vi "AnalogCNTL_Dakota3ch.vi"() -> ()   [LabVIEW 2015]
uses:
  <userlib>/caLab/Private/Put_DBL-1D_PV-1D.vi
  <vilib>/addons/control/pid/pid.llb/PID (DBL).vi
  <userlib>/caLab/Private/Get_PV-1D.vi
  <vilib>/addons/control/pid/NI_PID_pid.lvlib
  <vilib>/Analysis/NI_AALPro.lvlib
panel:
  out "APX:V7_SOP":bool
  out "APX:V7_SCL":bool
  in  "Gas_out_min_LIM":dbl min=0.0 max=1.0 step=0.02 format="%_3g"
  out "Error out":errorcluster
  out "APX:HPC":dbl format="%#_3g"
  out "APX:CellIn_MV":dbl
  out "APX:CellIn_MV2":dbl
  out "APX:CellIn_MV3":dbl
  out "Open 3":bool
  in  "Gas_in_min_LIM 3":dbl min=0.0 max=0.3 step=0.02 format="%_3g"
  in  "Gas_in_max_LIM 3":dbl min=0.0 max=2.0 step=0.02 format="%_3g"
  out "APX:CellIn_RV3":dbl(slide) scale=0.3..0.8
  out "slope OK":bool
  in  "slope loop":u8=15 min=10 max=30 step=1
  in  "Inlet2 offset":dbl
  out "APX:CellPressureState":u32
  in  "Threshold":dbl format="%#_13g"
  out "Inlet More":bool
  out "Open 2":bool
  in  "Gas_in_min_LIM 2":dbl min=0.0 max=0.3 step=0.02 format="%_3g"
  in  "Gas_in_max_LIM 2":dbl min=0.0 max=2.0 step=0.02 format="%_3g"
  out "APX:CellIn_RV2":dbl(slide) scale=0.3..0.8
  out "APX:CellOut_MV":dbl
  out "APX:OmniaxZ Failure":bool
  out "APX:CellMode":dbl
  out "APX:OmniaxZ":dbl
  out "APX:CellMode":bool
  out "PID_P":dbl format="%_4g"
  out "HPC Pressure Failure":bool
  out "HPC Turbo failure":bool
  out "<1.3":bool
  out "<2":bool
  out "OpenEx":bool
  out "APX:GAS":dbl format="%.2f"
  out "slope":dbl
  out "Open 1":bool
  in  "Inlet Mode":u16(ring) items=["Close", "Open", "Auto"]
  out "APX:CellIn_RV":sgl(slide)=0.8 min=0.3 max=0.8 step=0.05 scale=0.3..0.8
  out "Status":bool
  out "CellMode":u16
  out "Gas_out_max":dbl
  out "Period":i32
  out "Open Period":i32
  in  "Gas_in_min_LIM":dbl min=0.0 max=0.3 step=0.02 format="%_3g"
  in  "Gain":dbl=1.0 min=1.0 max=50.0 step=1.0 format="%_3g"
  in  "Gas_in_max_LIM":dbl=0.85 min=0.0 max=0.9 step=0.02 format="%_3g"
  in  "PID_D":dbl min=0.0 max=5.0 step=0.02 format="%_3g"
  in  "PID_I":dbl=0.5 min=0.005 max=5.0 step=0.02 format="%_3g"
  in  "PID_P_base":dbl=1.0 min=0.005 max=5.0 step=0.02 format="%_3g"
  in  "APX:CellPressure_RV":dbl=0.05 min=0.001 max=5.0 step=0.001 format="%.3f"
  out "PID_OC":dbl format="%.2f"
  out "PID dt out (s)":dbl format="%.3f"
  out "CellPressure":dbl(graph)
  in  "Exhasuet Mode":u16(ring) items=["Close", "Open", "Auto"]
  out "APX:AP1":dbl format="%#_3g"
  out "Outlet":sgl(slide)=2.0 min=0 max=5 step=0.05 scale=0.0..5.0
  out "APX:CellPressure_PV":dbl format="%_5g"
  in  "stop":bool
  # "Red LED ->\nClose-Close"
  # "if P>0.1 Period=Px100"
  # "Red LED ->\nClose-Open"
  # "Mk-II CH3"
  # "Ver 2023.12"
  # "0:Evacuate\n1: Auto-Auto\n2: Man-Man\n3: Man-Auto\n4: Auto-Man"
  # "Dakota 100000 sccm"
  # "8E-7 torr"
  # "record(ao, \"APX:CellIn_RV\")\n{\n    field(DESC, \"Double input without range infos\")\n    field(EGU, \"NA\")\n    field(PINI, \"YES\")\n}\nrecord(ao, \"APX:CellOut_RV\")\n{\n    field(DESC, \"Double input without range infos\")\n    field(EGU, \"NA\")\n    field(PINI, \"YES\")\n}\nrecord(ao, \"APX:CellIn_MV\")\n{\n    field(DESC, \"Double input without range infos\")\n    field(EGU, \"NA\")\n    field(PINI, \"YES\")\n}\nrecord(ao, \"APX:CellOut_MV\")\n{\n    field(DESC, \"Double input without range infos\")\n    field(EGU, \"NA\")\n    field(PINI, \"YES\")"
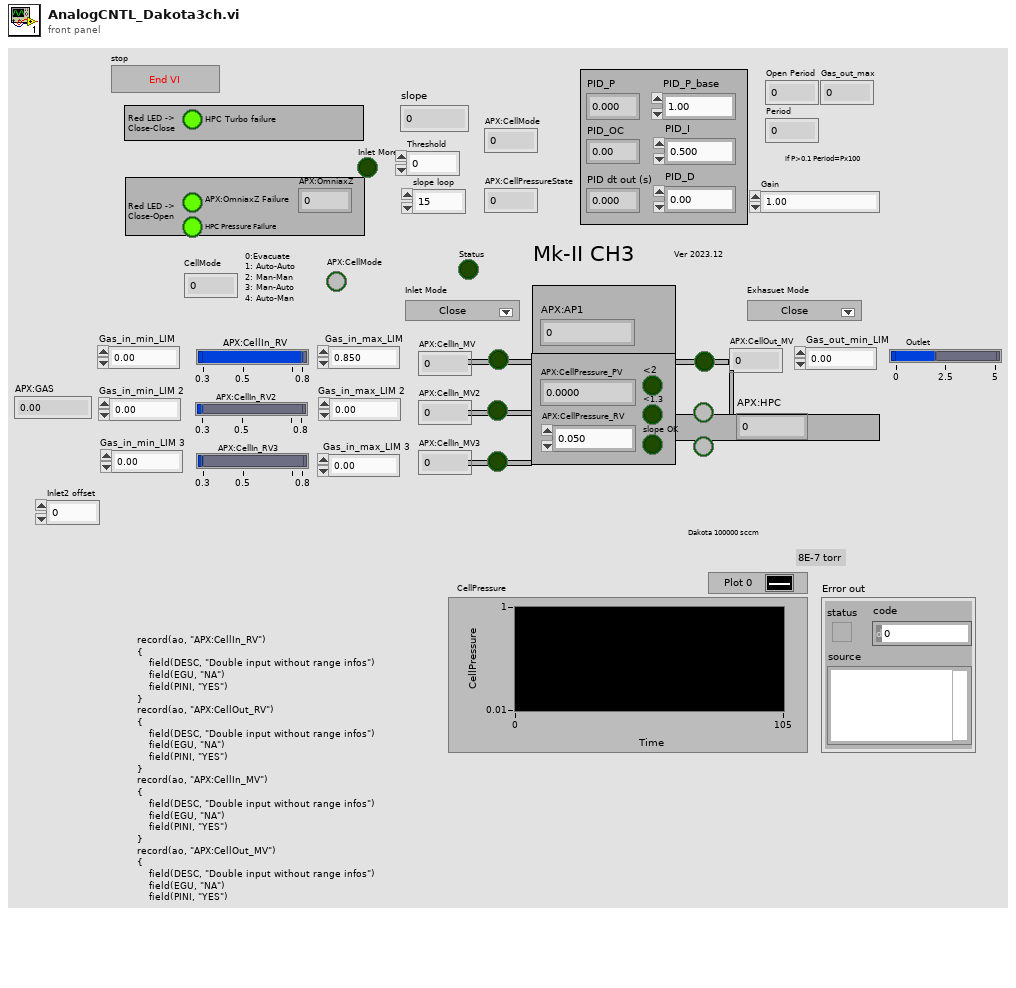
[diagram p1: front panel]
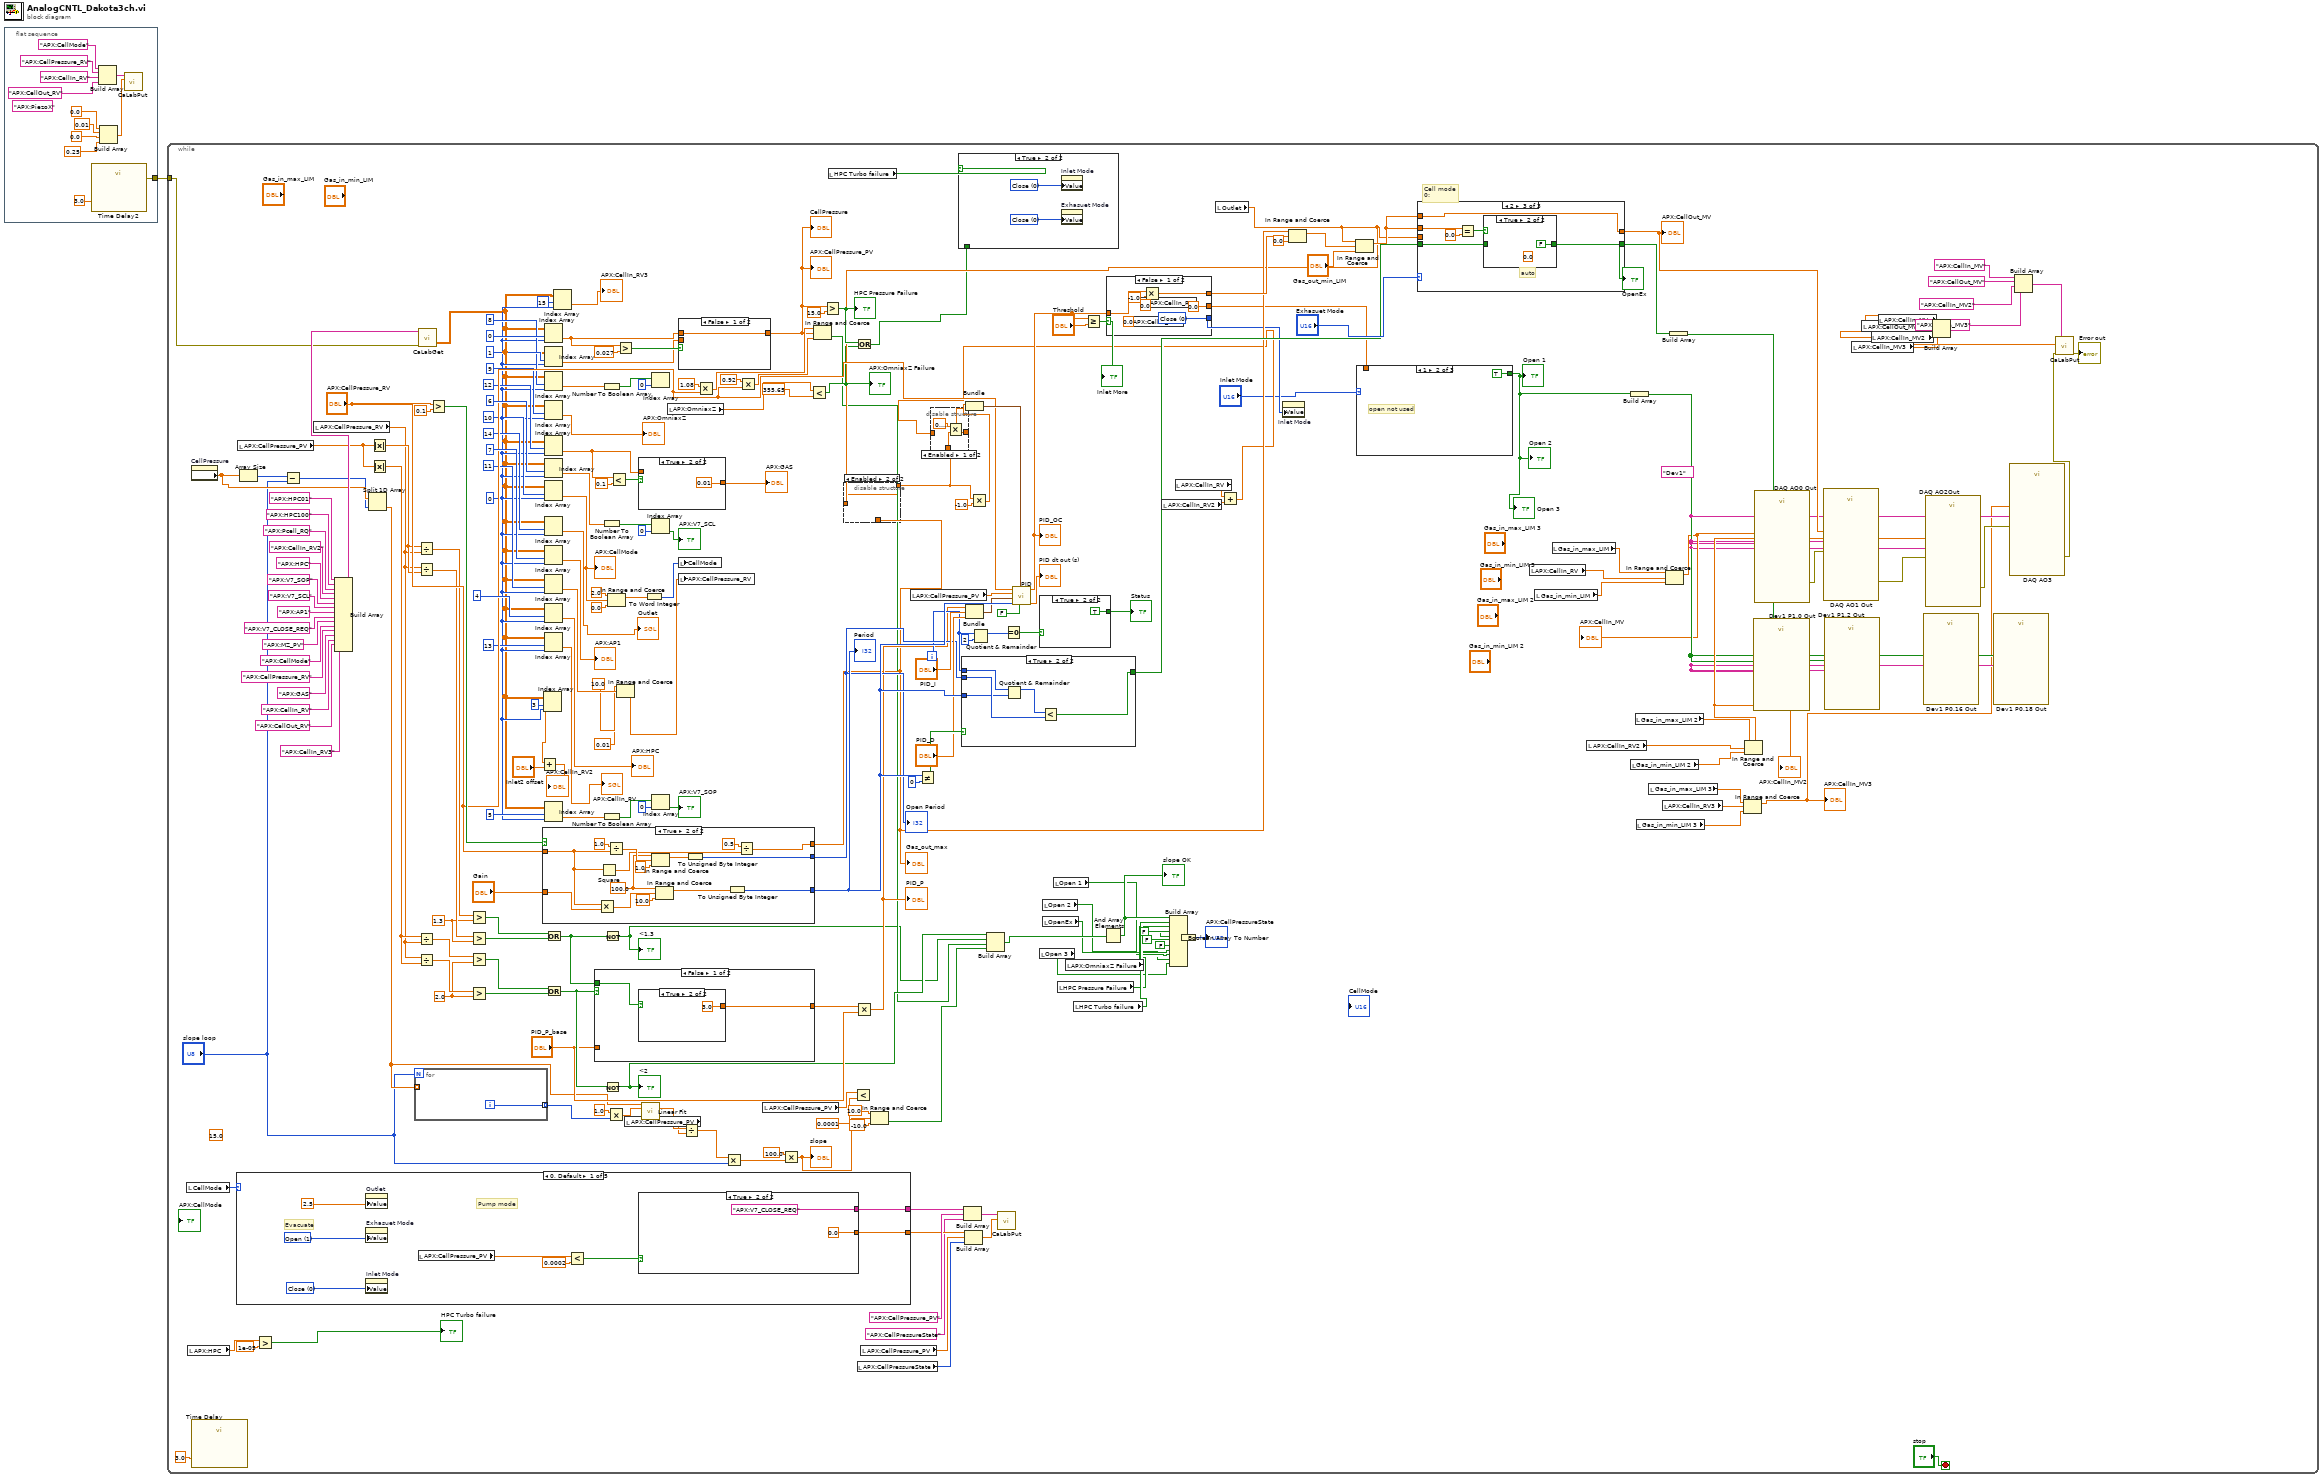
[diagram p0: block diagram]
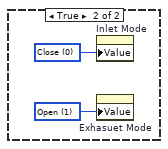
[diagram p6: hidden frame]
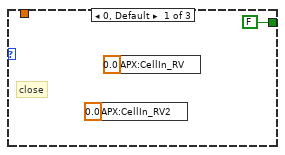
[diagram p7: hidden frame]
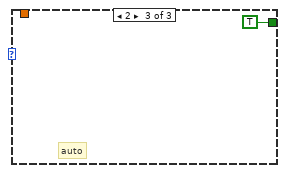
[diagram p8: hidden frame]
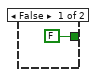
[diagram p9: hidden frame]
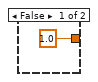
[diagram p10: hidden frame]
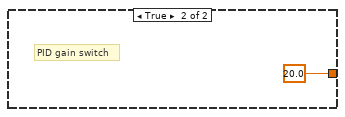
[diagram p11: hidden frame]
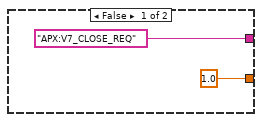
[diagram p12: hidden frame]
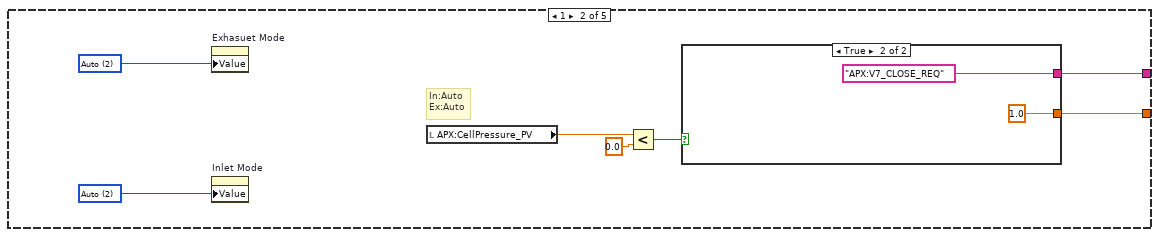
[diagram p13: hidden frame]
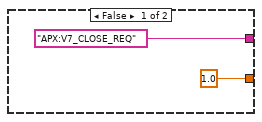
[diagram p14: hidden frame]
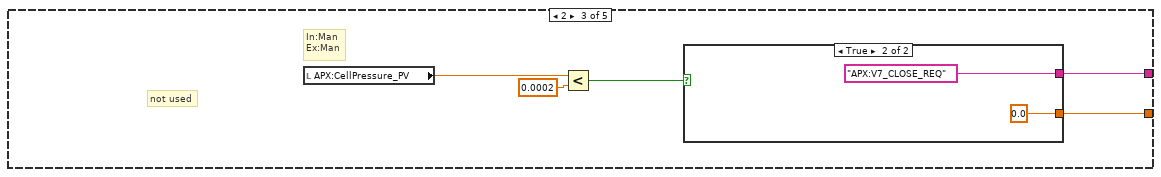
[diagram p15: hidden frame]
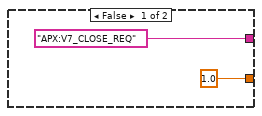
[diagram p16: hidden frame]
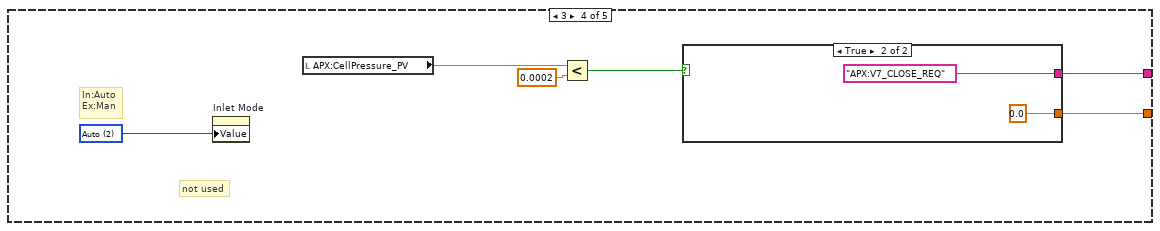
[diagram p17: hidden frame]
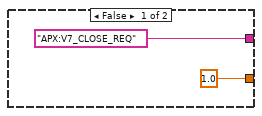
[diagram p18: hidden frame]
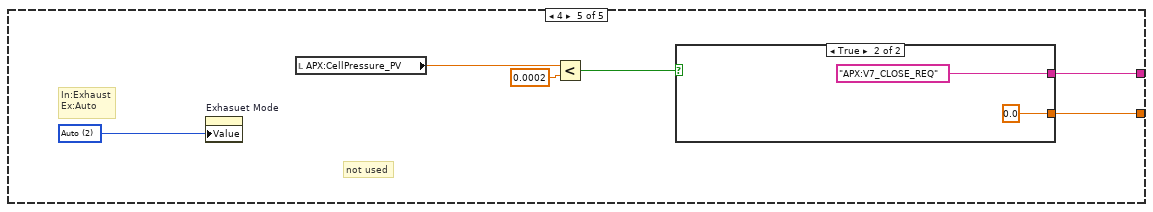
[diagram p19: hidden frame]
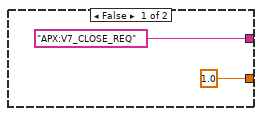
[diagram p20: hidden frame]
diagram:
  n1 = flat-sequence {
    tunnel: [w7] -> w1
    frame #0 {
      (unwired) "APX:PiezoX"
      n2 = call "Time Delay2"("Delay Time (s)"=3.0) -> ("error out"=w7:errorcluster)  [unwired: 10 in]
      n3 = Build Array("APX:CellMode", "APX:CellPressure_RV", "APX:CellIn_RV", "APX:CellOut_RV") -> (w11:string[])
      n4 = Build Array(0.0 ("element"), 0.01 ("element"), 0.0 ("element"), 0.25 ("element")) -> (w9:dbl[])
      n5 = call-poly <userlib>:"CaLabPut.vi"("Values"=w9, "PV Names"=w11) -> ()  [unwired: 6 in, 4 out]
    }
  }
  n6 = while {
    tunnel: w1 -> [w121]
    i -> [w176]
    stop <- "stop" stop-if-true
    w149 = 1.3 ("y")
    w158 = 2.0 ("y")
    (unwired) 15.0 ("y")
    w45 = 0 ("index (col)")
    w29 = tag "Dev1" ("device name")
    # "Cell mode \n0:"
    n7 = local read "CellMode"() -> (w111:u16)
    n8 = local read "APX:HPC"() -> (w139:dbl)
    n9 = property on="CellPressure" class="WFChart (strict)"() -> ("History Data"=w171:dbl[])  [unwired: 2 in, 2 out]
    n10 = call "Time Delay"("Delay Time (s)"=3.0) -> ()  [unwired: 10 in, 1 out]
    n11 = case shown="0, Default" w111 {
      tunnel: [w272 w283 w292 w302 w312] -> w127
      tunnel: [w271 w282 w291 w301 w311] -> w126
      frame 0, Default {
        w269 = u16 1 items=["Close", "Open", "Auto"] ("Exhasuet Mode")
        w270 = u16 0 items=["Close", "Open", "Auto"] ("Inlet Mod")
        # "Pump mode"
        # "Evacuate"
        n12 = property on="Outlet" class="Slide (strict)"("Value"=sgl 2.5 ("Exhaust")) -> ()  [unwired: 2 in, 2 out]
        n13 = property on="Exhasuet Mode" class="Ring (strict)"("Value"=w269) -> ()  [unwired: 2 in, 2 out]
        n14 = property on="Inlet Mode" class="Ring (strict)"("Value"=w270) -> ()  [unwired: 2 in, 2 out]
        n15 = local read "APX:CellPressure_PV"() -> (w267:dbl)
        n16 = Less?(x=w267, y=0.0002) -> (x < y?=w273:bool)
        n17 = case shown="True" w273 {
          tunnel: ["APX:V7_CLOSE_REQ" ("PV Name") "APX:V7_CLOSE_REQ" ("PV Name")] -> w272
          tunnel: [1.0 ("Value") 0.0 ("Value")] -> w271
          frame False {
          }
          frame True {
          }
        }
      }
      frame 1 {
        w280 = u16 2 items=["Close", "Open", "Auto"] ("Inlet Mod")
        w281 = u16 2 items=["Close", "Open", "Auto"] ("Exhasuet Mode")
        # "In:Auto\nEx:Auto"
        n18 = property on="Exhasuet Mode" class="Ring (strict)"("Value"=w281) -> ()  [unwired: 2 in, 2 out]
        n19 = property on="Inlet Mode" class="Ring (strict)"("Value"=w280) -> ()  [unwired: 2 in, 2 out]
        n20 = local read "APX:CellPressure_PV"() -> (w279:dbl)
        n21 = Less?(x=w279, y=0.0) -> (x < y?=w284:bool)
        n22 = case shown="True" w284 {
          tunnel: ["APX:V7_CLOSE_REQ" ("PV Name") "APX:V7_CLOSE_REQ" ("PV Name")] -> w283
          tunnel: [1.0 ("Value") 1.0 ("Value")] -> w282
          frame False {
          }
          frame True {
          }
        }
      }
      frame 2 {
        # "not used"
        # "In:Man\nEx:Man"
        n23 = local read "APX:CellPressure_PV"() -> (w290:dbl)
        n24 = Less?(x=w290, y=0.0002) -> (x < y?=w293:bool)
        n25 = case shown="True" w293 {
          tunnel: ["APX:V7_CLOSE_REQ" ("PV Name") "APX:V7_CLOSE_REQ" ("PV Name")] -> w292
          tunnel: [1.0 ("Value") 0.0 ("Value")] -> w291
          frame False {
          }
          frame True {
          }
        }
      }
      frame 3 {
        w300 = u16 2 items=["Close", "Open", "Auto"] ("Exhasuet Mode")
        # "not used"
        # "In:Auto\nEx:Man"
        n26 = property on="Inlet Mode" class="Ring (strict)"("Value"=w300) -> ()  [unwired: 2 in, 2 out]
        n27 = local read "APX:CellPressure_PV"() -> (w299:dbl)
        n28 = Less?(x=w299, y=0.0002) -> (x < y?=w303:bool)
        n29 = case shown="True" w303 {
          tunnel: ["APX:V7_CLOSE_REQ" ("PV Name") "APX:V7_CLOSE_REQ" ("PV Name")] -> w302
          tunnel: [1.0 ("Value") 0.0 ("Value")] -> w301
          frame False {
          }
          frame True {
          }
        }
      }
      frame 4 {
        w310 = u16 2 items=["Close", "Open", "Auto"] ("Exhasuet Mode")
        # "not used"
        # "In:Exhaust\nEx:Auto"
        n30 = property on="Exhasuet Mode" class="Ring (strict)"("Value"=w310) -> ()  [unwired: 2 in, 2 out]
        n31 = local read "APX:CellPressure_PV"() -> (w309:dbl)
        n32 = Less?(x=w309, y=0.0002) -> (x < y?=w313:bool)
        n33 = case shown="True" w313 {
          tunnel: ["APX:V7_CLOSE_REQ" ("PV Name") "APX:V7_CLOSE_REQ" ("PV Name")] -> w312
          tunnel: [1.0 ("Value") 0.0 ("Value")] -> w311
          frame False {
          }
          frame True {
          }
        }
      }
    }
    n34 = local read "APX:CellPressure_PV"() -> (w145:dbl)
    n35 = Array Size(array=w171) -> (size(s)=w169:i32)
    n36 = Greater?(x=w139, y=1e-05) -> (0:→"HPC Turbo failure":bool)
    n37 = Subtract(x=w169, y="slope loop") -> (x-y=w170:i32)
    n38 = local read "APX:CellPressure_RV"() -> (w144:dbl)
    n39 = Build Array("APX:HPC01", "APX:HPC100", "APX:Pcell_RQ", "APX:CellIn_RV2", "APX:HPC", "APX:V7_SOP", "APX:V7_SCL", "APX:AP1", "APX:V7_CLOSE_REQ", "APX:MZ_PV", "APX:CellMode", "APX:CellPressure_RV", "APX:GAS" ("element"), "APX:CellIn_RV", "APX:CellOut_RV", "APX:CellIn_RV3") -> (w239:string[])
    n40 = Split 1D Array(array=w171, index=w170) -> (second subarray=w73:dbl[])  [unwired: 1 out]
    n41 = Absolute Value(x=w145) -> (abs(x)=w146:dbl)
    n42 = Absolute Value(x=w145) -> (abs(x)=w152:dbl)
    n43 = for {
      N: "slope loop" -> [_]
      tunnel: w73 -> [_] mode=indexing
      tunnel: [w254] -> w168 mode=indexing
      i -> [w254]
    }
    n44 = Divide(x=w146, y=w144) -> (x/y=w151:dbl)
    n45 = Divide(x=w144, y=w146) -> (x/y=w150:dbl)
    n46 = Divide(x=w152, y=w144) -> (x/y=w160:dbl)
    n47 = Divide(x=w144, y=w152) -> (x/y=w159:dbl)
    n48 = call-poly "CaLabGet.vi"("PV Names"=w239, "Error in (no error)"=w121) -> ("Value Array (number)"=w43:dbl[][])  [unwired: 7 in, 6 out]
    n49 = Greater?(x="APX:CellPressure_RV", y=0.1) -> (0:w207:bool)
    n50 = Greater?(x=w151, y=w149) -> (0:w148:bool)
    n51 = Greater?(x=w150, y=w149) -> (0:w147:bool)
    n52 = Greater?(x=w160, y=w158) -> (0:w157:bool)
    n53 = Greater?(x=w159, y=w158) -> (0:w156:bool)
    n54 = case shown="True" w207 {
      tunnel: "APX:CellPressure_RV" -> [_ w332]
      tunnel: [w330 w341] -> w206
      tunnel: "Gain" -> [_ w345]
      tunnel: [w330 w335] -> w188
      tunnel: [5.0 w333] -> w87
      frame False {
        w330 = 10
      }
      frame True {
        w338 = 100.0 ("upper limit")
        n55 = Multiply(x=w332, y=w345) -> (x*y=w343:dbl)
        n56 = Square(x=w332) -> (x^2=w331:dbl)
        n57 = Divide(x=1.0, y=w332) -> (x/y=w339:dbl)
        n58 = In Range and Coerce(upper limit=w338, x=w339, lower limit=1.0) -> (coerced(x)=w336:dbl)  [unwired: 1 out]
        n59 = In Range and Coerce(upper limit=w338, x=w343, lower limit=10.0) -> (coerced(x)=w342:dbl)  [unwired: 1 out]
        n60 = To Unsigned Byte Integer(number=w336) -> (unsigned 8bit integer=w335:u8)
        n61 = To Unsigned Byte Integer(number=w342) -> (unsigned 8bit integer=w341:u8)
        n62 = Divide(x=0.5, y=w331) -> (x/y=w333:dbl)
      }
    }
    "Open Period" <- w188
    "Period" <- w206
    "Gas_out_max" <- w87
    n63 = Index Array(array=w43, index (row)=3, index (col)=w45) -> (element=w53:dbl)
    n64 = Add(x=w53, y="Inlet2 offset") -> (x+y=→"APX:CellIn_RV2":dbl)
    n65 = Index Array(array=w43, index (row)=1 ("disabled index (col)"), index (col)=w45) -> (element=w233:dbl)
    n66 = Index Array(array=w43, index (row)=8, index (col)=w45) -> (element=w184:dbl)
    n67 = Index Array(array=w43, index (row)=9 ("disabled index (row)"), index (col)=w45) -> (element=→"APX:OmniaxZ":dbl)
    n68 = Index Array(array=w43, index (row)=6, index (col)=w45) -> (element=w221:dbl)
    n69 = Index Array(array=w43, index (row)=14 ("disabled index (row)"), index (col)=w45) -> (element=→"Outlet":dbl)
    n70 = Index Array(array=w43, index (row)=7, index (col)=w45) -> (element=→"APX:AP1":dbl)
    n71 = Index Array(array=w43, index (row)=11, index (col)=w45) -> (element=w119:dbl)
    n72 = Index Array(array=w43, index (row)=4, index (col)=w45) -> (element=→"APX:HPC":dbl)
    n73 = Index Array(array=w43, index (row)=13 ("disabled index (row)"), index (col)=w45) -> (element=→"APX:CellIn_RV":dbl)
    n74 = Index Array(array=w43, index (row)=5, index (col)=w45) -> (element=w220:dbl)
    n75 = Index Array(array=w43, index (row)=0 ("disabled index (col)"), index (col)=w45) -> (element=w232:dbl)
    n76 = Index Array(array=w43, index (row)=12, index (col)=w45) -> (element=w103:dbl)
    n77 = Index Array(array=w43, index (row)=10, index (col)=w45) -> (element=w110:dbl)
    "APX:CellMode" <- w110
    n78 = Or(x=w148, y=w147) -> (x .or. y?=w143:bool)
    n79 = Or(x=w157, y=w156) -> (x .or. y?=w155:bool)
    n80 = Index Array(array=w43, index (row)=15, index (col)=w45) -> (element=→"APX:CellIn_RV3":dbl)
    n81 = case shown="False" w155 {
      tunnel: "PID_P_base" -> [_ _]
      tunnel: w143 -> [w263 _]
      tunnel: [w262 20.0 ("y")] -> w140
      frame False {
        n82 = case shown="True" w263 {
          tunnel: [1.0 ("y") 3.0 ("y")] -> w262
          frame False {
          }
          frame True {
          }
        }
      }
      frame True {
        # "PID gain switch"
      }
    }
    n83 = Number To Boolean Array(number=w184) -> (Boolean array=w183:bool[])
    n84 = Number To Boolean Array(number=w221) -> (Boolean array=w219:bool[])
    n85 = Number To Boolean Array(number=w220) -> (Boolean array=w216:bool[])
    n86 = Not(x=w143) -> (.not. x?=w51:bool)
    "<1.3" <- w51
    n87 = Not(x=w155) -> (.not. x?=w60:bool)
    "<2" <- w60
    n88 = Multiply(x=1.0, y=w168) -> (x*y=w167:dbl[])
    n89 = In Range and Coerce(upper limit=2.0, x=w110, lower limit=0.0) -> (coerced(x)=w112:dbl)  [unwired: 1 out]
    n90 = Less?(x=w103, y=0.1) -> (x < y?=w104:bool)
    n91 = Greater?(x=w232, y=0.027) -> (0:w235:bool)
    n92 = In Range and Coerce(upper limit=10.0, x=w119, lower limit=0.01) -> (coerced(x)=w116:dbl)  [unwired: 1 out]
    n93 = local read "APX:CellPressure_PV"() -> (w71:dbl)
    n94 = case shown="True" w104 {
      tunnel: w103 -> [w247 _]
      tunnel: [w247 0.01] -> w102
      frame False {
      }
      frame True {
      }
    }
    "APX:GAS" <- w102
    n95 = call <vilib>:"Linear Fit.vi"("Y"=w73, "X"=w167) -> ("slope"=w172:dbl)  [unwired: 9 in, 4 out]
    n96 = To Word Integer(number=w112) -> (16bit integer=w113:i16)
    n97 = Index Array(array=w183, index=0) -> ()  [unwired: 1 out]
    n98 = Index Array(array=w219, index=0) -> (element=→"APX:V7_SCL":bool)
    n99 = Index Array(array=w216, index=0) -> (element=→"APX:V7_SOP":bool)
    n100 = local read "APX:OmniaxZ"() -> (w62:dbl)
    n101 = case shown="False" w235 {
      tunnel: w233 -> [_ w371]
      tunnel: [w370 w371] -> w135
      tunnel: w232 -> [w370 _]
      frame False {
      }
      frame True {
      }
    }
    "APX:CellPressure_PV" <- w135
    "CellPressure" <- w135
    n102 = local write "CellMode"(w113) -> ()
    n103 = local write "APX:CellPressure_RV"(w116) -> ()
    n104 = Divide(x=w172, y=w71) -> (x/y=w162:dbl)
    n105 = Multiply(x=1.08, y="APX:CellPressure_RV") -> (x*y=w194:dbl)
    n106 = Multiply(x=w162, y="slope loop") -> (x*y=w161:dbl)
    n107 = Multiply(x=0.92, y="APX:CellPressure_RV") -> (x*y=w195:dbl)
    n108 = local read "APX:CellPressure_PV"() -> (w153:dbl)
    n109 = Multiply(x=100.0, y=w161) -> (x*y=w165:dbl)
    "slope" <- w165
    n110 = Less?(x=w62, y=355.65) -> (x < y?=w61:bool)
    "APX:OmniaxZ Failure" <- w61
    n111 = In Range and Coerce(upper limit=w194, x=w135, lower limit=w195) -> (In Range?=w59:bool)  [unwired: 1 out]
    n112 = Greater?(x=w135, y=15.0) -> (0:w134:bool)
    "HPC Pressure Failure" <- w134
    n113 = local read "HPC Turbo failure"() -> (w65:bool)
    n114 = Less?(x=w153, y=0.0001) -> ()  [unwired: 1 out]
    n115 = Or(x=w134, y=w61) -> (x .or. y?=w64:bool)
    n116 = Multiply(x=w140, y="PID_P_base") -> (x*y=w142:dbl)
    "PID_P" <- w142
    n117 = local read "APX:CellPressureState"() -> (w108:u32)
    n118 = local read "APX:CellPressure_PV"() -> (w123:dbl)
    n119 = In Range and Coerce(upper limit=10.0, x=w165, lower limit=-10.0) -> (In Range?=w58:bool)  [unwired: 1 out]
    n120 = local read "APX:CellPressure_PV"() -> (w186:dbl)
    n121 = Not Equal?(x=w206, y=u8 0) -> (x != y?=w212:bool)
    n122 = case shown="True" w65 {
      tunnel: w64 -> [w249 _]
      frame False {
        n123 = case shown="False" w249 {
          frame False {
          }
          frame True {
            w250 = u16 1 items=["Close", "Open", "Auto"] ("Inlet Mod")
            w251 = u16 0 items=["Close", "Open", "Auto"] ("Exhasuet Mode")
            n124 = property on="Inlet Mode" class="Ring (strict)"("Value"=w251) -> ()  [unwired: 2 in, 2 out]
            n125 = property on="Exhasuet Mode" class="Ring (strict)"("Value"=w250) -> ()  [unwired: 2 in, 2 out]
          }
        }
      }
      frame True {
        w252 = u16 0 items=["Close", "Open", "Auto"] ("Inlet Mod")
        w253 = u16 0 items=["Close", "Open", "Auto"] ("Exhasuet Mode")
        n126 = property on="Inlet Mode" class="Ring (strict)"("Value"=w253) -> ()  [unwired: 2 in, 2 out]
        n127 = property on="Exhasuet Mode" class="Ring (strict)"("Value"=w252) -> ()  [unwired: 2 in, 2 out]
      }
    }
    n128 = case shown="True" w212 {
      tunnel: w176 -> [_ w369]
      tunnel: [FALSE w368] -> w173
      tunnel: w206 -> [_ w365]
      tunnel: w188 -> [_ w367]
      frame False {
      }
      frame True {
        n129 = Quotient & Remainder(x=w369, y=w365) -> (x-y*floor(x/y)=w366:i32)  [unwired: 1 out]
        n130 = Less?(x=w366, y=w367) -> (x < y?=w368:bool)
      }
    }
    n131 = Build Array(w127, "APX:CellPressure_PV", "APX:CellPressureState") -> (w124:string[])
    n132 = Build Array(w126, w123, w108) -> (w125:dbl[])
    n133 = Bundle(w142, "PID_I"="PID_I", "PID_D"="PID_D") -> (w202:cluster{dbl, "PID_I":dbl, "PID_D":dbl})  [unwired: 1 in]
    n134 = Quotient & Remainder(x=w176, y=2) -> (x-y*floor(x/y)=w179:i32)  [unwired: 1 out]
    n135 = Build Array(w60, w51, w59, w58) -> (w57:bool[])
    n136 = call-poly <userlib>:"CaLabPut.vi"("Values"=w125, "PV Names"=w124) -> ()  [unwired: 6 in, 4 out]
    n137 = Equal To 0?(x=w179) -> (x = 0?=w180:bool)
    n138 = case shown="True" w180 {
      tunnel: [FALSE ("Status") TRUE ("Status")] -> w177
      frame False {
      }
      frame True {
      }
    }
    "Status" <- w177
    n139 = local read "Open 3"() -> (w16:bool)
    n140 = local read "Open 2"() -> (w17:bool)
    n141 = local read "OpenEx"() -> (w19:bool)
    n142 = local read "Open 1"() -> (w18:bool)
    n143 = local read "HPC Pressure Failure"() -> (w23:bool)
    n144 = local read "APX:OmniaxZ Failure"() -> (w24:bool)
    n145 = local read "HPC Turbo failure"() -> (w25:bool)
    n146 = And Array Elements(Boolean array=w57) -> (logical AND=w47:bool)
    "slope OK" <- w47
    n147 = local read "APX:CellIn_RV2"() -> (w75:dbl)
    n148 = Build Array(w47, w25, w24, w23, FALSE ("element"), FALSE ("element"), FALSE ("element"), w19, w18, w17, w16) -> (w56:bool[])
    n149 = local read "APX:CellIn_RV"() -> (w74:sgl)
    n150 = Boolean Array To Number(Boolean array=w56) -> (number=→"APX:CellPressureState":u32)
    n151 = local read "Outlet"() -> (w70:sgl)
    n152 = disable-structure shown="Enabled" {
      disable-tunnel: w87 -> [w245 _]
      disable-tunnel: [w245 w246] -> w67
      disable-tunnel: w70 -> [_ w246]
      frame Disabled {
      }
      frame Enabled {
      }
    }
    n153 = Multiply(x=w67, y=-1.0) -> (x*y=w86:dbl)
    n154 = Add(x=w74, y=w75) -> (x+y=w69:dbl)
    n155 = disable-structure shown="Enabled" {
      disable-tunnel: w69 -> [_ _]
      disable-tunnel: [w243 _] -> w68
      disable-tunnel: w67 -> [w244 _]
      frame Enabled {
        n156 = Multiply(x=sgl 0.1, y=w244) -> (x*y=w243:sgl)
      }
      frame Disabled {
      }
    }
    n157 = Bundle(w86, w68) -> (w199:cluster{dbl, sgl})  [unwired: 1 in]
    n158 = call-poly <vilib>:"PID.vi"("reinitialize? (F)"=FALSE, "output range"=w199, "dt (s)"=w206, "PID gains"=w202, "process variable"=w186, "setpoint"="APX:CellPressure_RV") -> ("dt out (s)"=→"PID dt out (s)":dbl, "output"=w189:dbl)  [unwired: 4 in]
    "PID_OC" <- w189
    n159 = Greater Or Equal?(x=w189, y="Threshold") -> (x >= y?=w197:bool)
    "Inlet More" <- w197
    n160 = case shown="False" w197 {
      tunnel: [w324 0.0] -> w190
      tunnel: w189 -> [w325 w327]
      tunnel: [0.0 w327] -> w66
      tunnel: [w321 w326] -> w50
      frame False {
        w321 = u16 0 items=["Close", "Open", "Auto"] ("Inlet Mode")
        n161 = local write "APX:CellIn_RV2"(0.0 ("Inlet2")) -> ()
        n162 = local write "APX:CellIn_RV"(sgl 0.0 ("Inlet")) -> ()
        n163 = Multiply(x=w325, y=-1.0) -> (x*y=w324:dbl)
      }
      frame True {
        w326 = u16 2 items=["Close", "Open", "Auto"] ("Inlet Mode")
      }
    }
    n164 = property on="Inlet Mode" class="Ring (strict)"("Value"=w50) -> ()  [unwired: 2 in, 2 out]
    n165 = In Range and Coerce(upper limit=w87, x=w190, lower limit=0.0) -> (coerced(x)=w89:dbl)  [unwired: 1 out]
    n166 = In Range and Coerce(upper limit=w70, x=w89, lower limit="Gas_out_min_LIM") -> (coerced(x)=w88:dbl)  [unwired: 1 out]
    n167 = case shown="1" "Inlet Mode" {
      tunnel: [FALSE TRUE TRUE] -> w41
      tunnel: w66 -> [_ _ _]
      frame 0, Default {
        # "close"
        n168 = local write "APX:CellIn_RV2"(0.0 ("Inlet2")) -> ()
        n169 = local write "APX:CellIn_RV"(sgl 0.0 ("Inlet")) -> ()
      }
      frame 1 {
        # "open not used"
      }
      frame 2 {
        # "auto"
      }
    }
    "Open 1" <- w41
    "Open 2" <- w41
    "Open 3" <- w41
    n170 = case shown="2" "Exhasuet Mode" {
      tunnel: w173 -> [_ w351 w357]
      tunnel: [0.0 2.5 ("y") w361] -> w175
      tunnel: w88 -> [_ _ w361]
      tunnel: w88 -> [_ _ w360]
      tunnel: w70 -> [_ w349 _]
      tunnel: [FALSE w350 w356] -> w90
      frame 0, Default {
        # "Close"
      }
      frame 1 {
        # "open"
        n171 = Equal?(x=w349, y=0.0) -> (x = y?=w352:bool)
        n172 = case shown="True" w352 {
          tunnel: w351 -> [_ _]
          tunnel: [TRUE TRUE] -> w350
          frame False {
          }
          frame True {
          }
        }
      }
      frame 2 {
        # "auto"
        n173 = Equal?(x=w360, y=0.0) -> (x = y?=w358:bool)
        n174 = case shown="True" w358 {
          tunnel: w357 -> [w362 _]
          tunnel: [w362 FALSE] -> w356
          frame False {
          }
          frame True {
            (unwired) 0.0
          }
        }
      }
    }
    "OpenEx" <- w90
    "APX:CellOut_MV" <- w175
    n175 = local read "APX:CellIn_RV"() -> (w82:sgl)
    n176 = local read "Gas_in_min_LIM"() -> (w33:dbl)
    n177 = local read "Gas_in_max_LIM"() -> (w32:dbl)
    n178 = local read "APX:CellIn_RV2"() -> (w81:dbl)
    n179 = local read "Gas_in_min_LIM 2"() -> (w78:dbl)
    n180 = Build Array(w41) -> (w35:bool[])
    n181 = local read "Gas_in_max_LIM 2"() -> (w79:dbl)
    n182 = local read "Gas_in_min_LIM 3"() -> (w37:dbl)
    n183 = local read "Gas_in_max_LIM 3"() -> (w38:dbl)
    n184 = local read "APX:CellIn_RV3"() -> (w39:dbl)
    n185 = In Range and Coerce(upper limit=w32, x=w82, lower limit=w33) -> (coerced(x)=w34:dbl)  [unwired: 1 out]
    "APX:CellIn_MV" <- w34
    n186 = Build Array(w90) -> (w174:bool[])
    n187 = In Range and Coerce(upper limit=w38, x=w39, lower limit=w37) -> (coerced(x)=w28:dbl)  [unwired: 1 out]
    "APX:CellIn_MV3" <- w28
    n188 = In Range and Coerce(upper limit=w79, x=w81, lower limit=w78) -> (coerced(x)=w80:dbl)  [unwired: 1 out]
    "APX:CellIn_MV2" <- w80
    n189 = call "Dev1 P1.0 Out"("data"=w35, "device name"=w29) -> ()  [unwired: 16 in, 2 out]
    n190 = call "DAQ AO0 Out"("data"=w34, "device name"=w29) -> ("error out"=w93:errorcluster)  [unwired: 16 in, 1 out]
    n191 = call "DAQ AO1 Out"("data"=w175, "error in"=w93, "device name"=w29) -> ("error out"=w31:errorcluster)  [unwired: 15 in, 1 out]
    n192 = call "Dev1 P1.2 Out"("data"=w174, "device name"=w29) -> ()  [unwired: 16 in, 2 out]
    n193 = local read "APX:CellIn_MV3"() -> (w36:dbl)
    n194 = local read "APX:CellOut_MV"() -> (w91:dbl)
    n195 = local read "APX:CellIn_MV2"() -> (w76:dbl)
    n196 = local read "APX:CellIn_MV"() -> (w92:dbl)
    n197 = call "Dev1 P0.16 Out"("data"=w35, "device name"=w29) -> ()  [unwired: 16 in, 2 out]
    n198 = call "DAQ AO2Out"("data"=w80, "error in"=w31, "device name"=w29) -> ("error out"=w30:errorcluster)  [unwired: 15 in, 1 out]
    n199 = Build Array(w92, w91, w76, w36) -> (w94:dbl[])
    n200 = call "Dev1 P0.18 Out"("data"=w35, "device name"=w29) -> ()  [unwired: 16 in, 2 out]
    n201 = call "DAQ AO3"("data"=w28, "error in"=w30, "device name"=w29) -> ("error out"=w27:errorcluster)  [unwired: 15 in, 1 out]
    n202 = Build Array("APX:CellIn_MV", "APX:CellOut_MV", "APX:CellIn_MV2", "APX:CellIn_MV3") -> (w95:string[])
    n203 = call-poly <userlib>:"CaLabPut.vi"("Error in (no error)"=w27, "Values"=w94, "PV Names"=w95) -> ("Error out"=→"Error out":errorcluster)  [unwired: 5 in, 3 out]
  }
